vi "HTTP Request.vi"(0 "REST Client in":refnum<class "REST Client.lvclass">, 1 "Request body":string, 2 "Multipart Post data":T1[](array[typedef]), 5 "Method":T2, 9 "Path":string, 11 "error in (no error)":errorcluster, 12 "request specific headers":T3[](array[typedef]), 13 "timeout (0 = Use Default)":i32) -> (3 "Status Code":u16, 4 "REST Client out":refnum<class "REST Client.lvclass">, 6 "Response Headers out":refnum<class "Response Headers.lvclass">, 10 "Response body":string, 14 "Status String":string, 15 "error out":errorcluster)   [LabVIEW 2020, in "REST Client.lvlib" / "REST Client.lvclass"]
uses:
  REST Client.lvclass
  Response Headers/Response Headers.lvclass
  HTTP Header.ctl
  HTTP Methods.ctl
  <vilib>/httpClient/MultipartData.ctl
  <vilib>/NI/Advanced HTTP Client/Multipart Data--cluster.ctl
  <vilib>/VIPM Community/HTTP Client Plugin - Base/Classes/Abstract HTTP Client/Abstract HTTP Client.lvclass
  <vilib>/NI/Advanced HTTP Client/Session.lvclass
  http-client/http-client.lvclass
  <vilib>/httpClient/LabVIEWHTTPClient.lvlib
panel:
  # "Copyright © 2014 JKI All rights reserved.\n\nAuthor: Tomi Maila <tomi.maila@jki.net>\n\nThis library is provided \"AS IS\" ,WITHOUT WARRANTIES OR \nCONDITIONS OF ANY KIND, either express or implied.\n\nJKI -- jki.net"
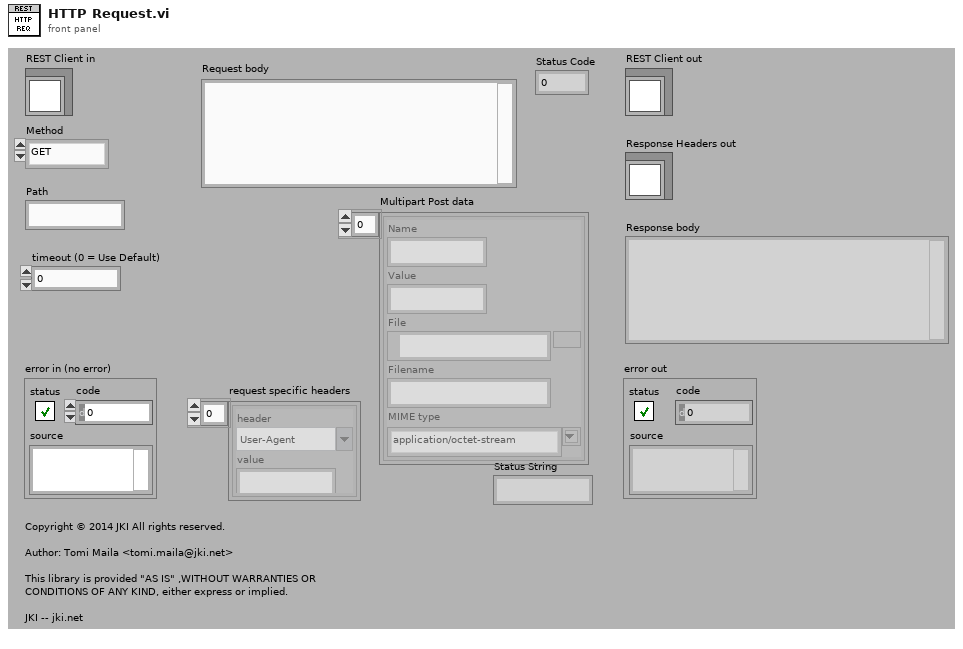
[diagram p1: front panel]
types:
  T1 = typedef "LabVIEWHTTPClient.lvlib/MultipartData.ctl" = cluster{"Name":string, "Value":string, "File":path, "Filename":string, "MIME type":string}
  T2 = typedef "REST Client.lvlib/REST Client.lvclass/HTTP Methods.ctl" = enum16{"GET", "HEAD", "POST", "PUT", "DELETE", "PATCH"}
  T3 = typedef "REST Client.lvlib/REST Client.lvclass/HTTP Header.ctl" = cluster{"header":string, "value":string}
  T4 = typedef "lib_NI_Advanced HTTP Client.lvlib/Session.lvclass/Multipart Data--cluster.ctl" = cluster{"name":string, "value":string, "file":path, "filename":string, "MIME type":string}
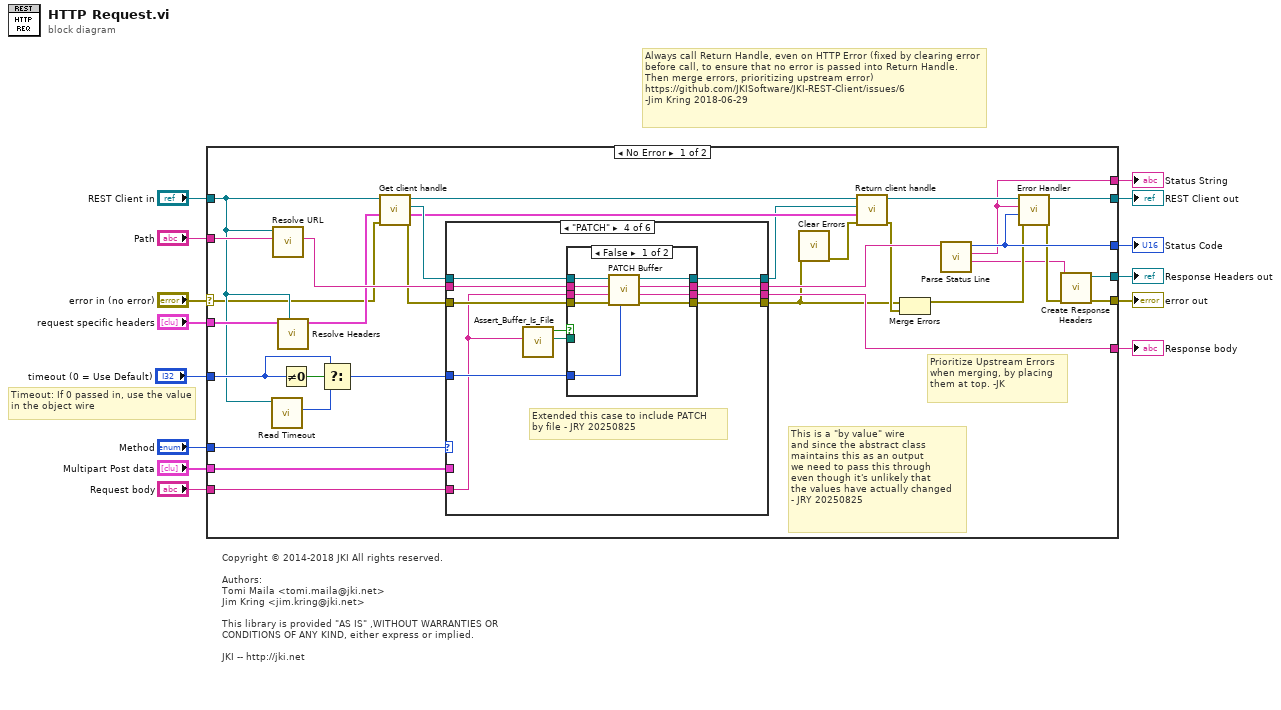
[diagram p0: block diagram]
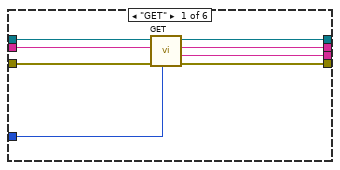
[diagram p2: hidden frame]
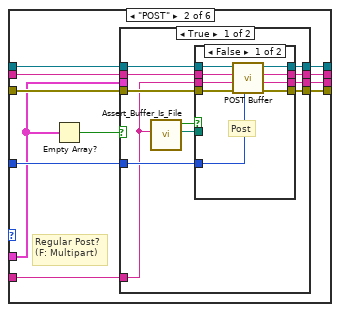
[diagram p3: hidden frame]
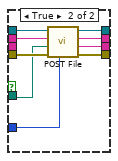
[diagram p4: hidden frame]
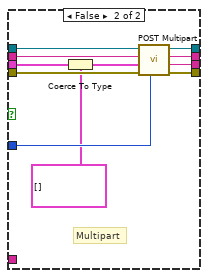
[diagram p5: hidden frame]
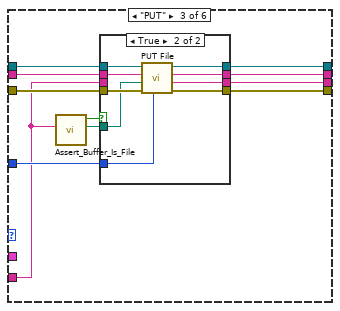
[diagram p6: hidden frame]
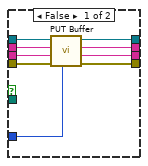
[diagram p7: hidden frame]
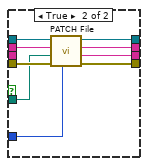
[diagram p8: hidden frame]
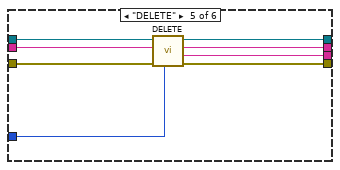
[diagram p9: hidden frame]
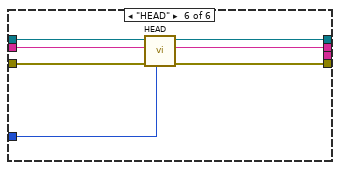
[diagram p10: hidden frame]
diagram:
  # "Always call Return Handle, even on HTTP Error (fixed by clearing error before call, to ensure that no error is passed into Return Handle. Then merge errors, prioritizing upstream error)\nhttps://github.com/JKISoftware/JKI-REST-Client/issues/6\n-Jim Kring 2018-06-29"
  # "Timeout: If 0 passed in, use the value in the object wire"
  # "Copyright © 2014-2018 JKI All rights reserved.\n\nAuthors:\nTomi Maila <tomi.maila@jki.net>\nJim Kring <jim.kring@jki.net>\n\nThis library is provided \"AS IS\" ,WITHOUT WARRANTIES OR \nCONDITIONS OF ANY KIND, either express or implied.\n\nJKI -- http://jki.net"
  n1 = case shown="No Error" "error in (no error)" {
    selector: "error in (no error)" -> [w15 w180]
    tunnel: [w34 w180] -> w13
    tunnel: [w41 w179] -> w11
    tunnel: "REST Client in" -> [w16 w179]
    tunnel: "Method" -> [w40 _]
    tunnel: "Path" -> [w39 _]
    tunnel: "Request body" -> [w26 _]
    tunnel: [w21 _] -> w8
    tunnel: [w35 _] -> w3
    tunnel: [w37 _] -> w7
    tunnel: "request specific headers" -> [w18 _]
    tunnel: [w36 _] -> w4
    tunnel: "Multipart Post data" -> [w33 _]
    tunnel: "timeout (0 = Use Default)" -> [w28 _]
    frame No Error {
      # "This is a \"by value\" wire\nand since the abstract class\nmaintains this as an output\nwe need to pass this through\neven though it's unlikely that\nthe values have actually changed\n- JRY 20250825"
      # "Prioritize Upstream Errors when merging, by placing them at top. -JK"
      n2 = call-dynamic "Read Timeout.vi"("REST Client in"=w16) -> ("Timeout"=w24:i32)  [unwired: 8 in, 2 out]
      n3 = call "Resolve URL.vi"("Path"=w39, "REST Client in"=w16) -> ("Resolved URL"=w38:string)  [unwired: 9 in]
      n4 = call "Resolve Headers.vi"("REST Client in"=w16, "headers in"=w18) -> ("headers out"=w17:T3[])  [unwired: 9 in]
      n5 = Not Equal To 0?(x=w28) -> (x != 0?=w29:bool)
      n6 = Select(t=w28, s=w29, f=w24) -> (s? t:f=w27:i32)
      n7 = call "Get client handle.vi"("error in (no error)"=w15, "headers"=w17, "REST Client in"=w16) -> ("error out"=w25:errorcluster, "headers out"=w43:T3[], "Client Handle"=w44:refnum<class "Abstract HTTP Client.lvclass">, "REST Client out"=w45:refnum<class "REST Client.lvclass">)  [unwired: 5 in]
      n8 = case shown="\"PATCH\"" w40 {
        tunnel: w38 -> [w53 w65 w116 w141 w166 w175]
        tunnel: w27 -> [w48 w64 w115 w142 w165 w177]
        tunnel: w25 -> [w52 w63 w114 w140 w170 w178]
        tunnel: [w49 w62 w113 w137 w167 w173] -> w46
        tunnel: [w50 w61 w112 w136 w168 _] -> w37
        tunnel: [w51 w60 w111 w135 w169 w176] -> w31
        tunnel: w44 -> [w54 w59 w110 w143 w171 w174]
        tunnel: w33 -> [_ w57 _ _ _ _]
        tunnel: w26 -> [_ w56 w109 w139 _ _]
        tunnel: [w47 w55 w106 w138 w164 w172] -> w19
        frame "GET" {
          n9 = call-dynamic "GET.vi"("timeout (10000)"=w48, "error in (no error)"=w52, "url"=w53, "HTTP Client Abstract in"=w54) -> ("error out"=w51:errorcluster, "body"=w50:string, "headers"=w49:string, "HTTP Client Abstract out"=w47:refnum<class "Abstract HTTP Client.lvclass">)  [unwired: 3 in, 1 out]
        }
        frame "POST" {
          # "Regular Post?\n(F: Multipart)"
          n10 = Empty Array?(array=w57) -> (empty?=w58:bool)
          n11 = case shown="True" w58 {
            tunnel: w65 -> [w76 w104]
            tunnel: w64 -> [w75 w99]
            tunnel: w63 -> [w74 w103]
            tunnel: [w73 w102] -> w62
            tunnel: [w72 w101] -> w61
            tunnel: [w71 w100] -> w60
            tunnel: w59 -> [w70 w105]
            tunnel: w56 -> [w69 _]
            tunnel: w57 -> [_ w96]
            tunnel: [w66 w95] -> w55
            frame True {
              n12 = call "Assert_Buffer_Is_File.vi"("body"=w69) -> ("File"=w67:path, "is File?"=w68:bool)  [unwired: 9 in]
              n13 = case shown="False" w68 {
                tunnel: w76 -> [w78 w89]
                tunnel: w75 -> [w81 w87]
                tunnel: w74 -> [w80 w90]
                tunnel: [w84 w93] -> w73
                tunnel: [w83 w92] -> w72
                tunnel: [w82 w91] -> w71
                tunnel: w70 -> [w85 w94]
                tunnel: w69 -> [w79 _]
                tunnel: w67 -> [_ w88]
                tunnel: [w77 w86] -> w66
                frame False {
                  # "Post"
                  n14 = call-dynamic "POST Buffer.vi"("timeout (10000)"=w81, "error in (no error)"=w80, "buffer"=w79, "url"=w78, "HTTP Client Abstract in"=w85) -> ("error out"=w82:errorcluster, "body"=w83:string, "headers"=w84:string, "HTTP Client Abstract out"=w77:refnum<class "Abstract HTTP Client.lvclass">)  [unwired: 2 in, 1 out]
                }
                frame True {
                  n15 = call-dynamic "POST File.vi"("timeout (10000)"=w87, "error in (no error)"=w90, "file"=w88, "url"=w89, "HTTP Client Abstract in"=w94) -> ("error out"=w91:errorcluster, "body"=w92:string, "headers"=w93:string, "HTTP Client Abstract out"=w86:refnum<class "Abstract HTTP Client.lvclass">)  [unwired: 2 in, 1 out]
                }
              }
            }
            frame False {
              # "Multipart"
              n16 = Coerce To Type(0:w96, 1:T4[] [] ("Multipart Post data")) -> (2:w97:T4[])
              n17 = call-dynamic "POST Multipart.vi"("timeout (10000)"=w99, "error in (no error)"=w103, "data"=w97, "url"=w104, "HTTP Client Abstract in"=w105) -> ("error out"=w100:errorcluster, "body"=w101:string, "headers"=w102:string, "HTTP Client Abstract out"=w95:refnum<class "Abstract HTTP Client.lvclass">)  [unwired: 2 in, 1 out]
            }
          }
        }
        frame "PUT" {
          n18 = call "Assert_Buffer_Is_File.vi"("body"=w109) -> ("File"=w107:path, "is File?"=w108:bool)  [unwired: 9 in]
          n19 = case shown="True" w108 {
            tunnel: w116 -> [w124 w127]
            tunnel: w115 -> [w121 w128]
            tunnel: w114 -> [w122 w133]
            tunnel: [w118 w130] -> w113
            tunnel: [w119 w131] -> w112
            tunnel: [w120 w132] -> w111
            tunnel: w110 -> [w125 w134]
            tunnel: w109 -> [w123 _]
            tunnel: w107 -> [_ w129]
            tunnel: [w117 w126] -> w106
            frame False {
              n20 = call-dynamic "PUT Buffer.vi"("timeout (10000)"=w121, "error in (no error)"=w122, "buffer"=w123, "url"=w124, "HTTP Client Abstract in"=w125) -> ("error out"=w120:errorcluster, "body"=w119:string, "headers"=w118:string, "HTTP Client Abstract out"=w117:refnum<class "Abstract HTTP Client.lvclass">)  [unwired: 2 in, 1 out]
            }
            frame True {
              n21 = call-dynamic "PUT File.vi"("timeout (10000)"=w128, "error in (no error)"=w133, "file"=w129, "url"=w127, "HTTP Client Abstract in"=w134) -> ("error out"=w132:errorcluster, "body"=w131:string, "headers"=w130:string, "HTTP Client Abstract out"=w126:refnum<class "Abstract HTTP Client.lvclass">)  [unwired: 2 in, 1 out]
            }
          }
        }
        frame "PATCH" {
          # "Extended this case to include PATCH\nby file - JRY 20250825"
          n22 = call "Assert_Buffer_Is_File.vi"("body"=w139) -> ("File"=w144:path, "is File?"=w145:bool)  [unwired: 9 in]
          n23 = case shown="False" w145 {
            tunnel: w141 -> [w153 w156]
            tunnel: w142 -> [w150 w157]
            tunnel: w140 -> [w151 w162]
            tunnel: [w147 w159] -> w137
            tunnel: [w148 w160] -> w136
            tunnel: [w149 w161] -> w135
            tunnel: w143 -> [w154 w163]
            tunnel: w139 -> [w152 _]
            tunnel: w144 -> [_ w158]
            tunnel: [w146 w155] -> w138
            frame False {
              n24 = call-dynamic "PATCH Buffer.vi"("timeout"=w150, "error in (no error)"=w151, "buffer"=w152, "url"=w153, "HTTP Client Abstract in"=w154) -> ("error out"=w149:errorcluster, "body"=w148:string, "headers"=w147:string, "HTTP Client Abstract out"=w146:refnum<class "Abstract HTTP Client.lvclass">)  [unwired: 2 in, 1 out]
            }
            frame True {
              n25 = call-dynamic "PATCH File.vi"("timeout"=w157, "error in (no error)"=w162, "file"=w158, "url"=w156, "HTTP Client Abstract in"=w163) -> ("error out"=w161:errorcluster, "body"=w160:string, "headers"=w159:string, "HTTP Client Abstract out"=w155:refnum<class "Abstract HTTP Client.lvclass">)  [unwired: 2 in, 1 out]
            }
          }
        }
        frame "DELETE" {
          n26 = call-dynamic "DELETE.vi"("timeout (10000)"=w165, "error in (no error)"=w170, "url"=w166, "HTTP Client Abstract in"=w171) -> ("error out"=w169:errorcluster, "body"=w168:string, "headers"=w167:string, "HTTP Client Abstract out"=w164:refnum<class "Abstract HTTP Client.lvclass">)  [unwired: 3 in, 1 out]
        }
        frame "HEAD" {
          n27 = call-dynamic "HEAD.vi"("timeout (10000)"=w177, "error in (no error)"=w178, "url"=w175, "HTTP Client Abstract in"=w174) -> ("error out"=w176:errorcluster, "headers"=w173:string, "HTTP Client Abstract out"=w172:refnum<class "Abstract HTTP Client.lvclass">)  [unwired: 4 in, 1 out]
        }
      }
      n28 = call <vilib>:"Clear Errors.vi"("error in (no error)"=w31) -> ("error out"=w30:errorcluster)  [unwired: 5 in, 1 out]
      n29 = call "Return client handle.vi"("error in (no error)"=w30, "headers"=w43, "Client Handle"=w19, "REST Client in"=w45) -> ("error out"=w32:errorcluster, "REST Client out"=w42:refnum<class "REST Client.lvclass">)  [unwired: 6 in]
      n30 = Merge Errors(w31, w32) -> (w22:errorcluster)
      n31 = call "Parse Status Line.vi"("Headers w/ status line"=w46) -> ("HTTP Headers"=w20:string, "Status String"=w21:string, "status code"=w36:u16)  [unwired: 6 in, 2 out]
      n32 = call-dynamic "Error Handler.vi"("error in (no error)"=w22, "Status Code"=w36, "Status String"=w21, "REST Client in"=w42) -> ("error out"=w23:errorcluster, "REST Client out"=w41:refnum<class "REST Client.lvclass">)  [unwired: 6 in]
      n33 = call "Create Response Headers.vi"("error in (no error)"=w23, "Response Headers"=w20) -> ("error out"=w34:errorcluster, "Response Headers out"=w35:refnum<class "Response Headers.lvclass">)  [unwired: 8 in]
    }
    frame Error {
    }
  }
  "error out" <- w13
  "REST Client out" <- w11
  "Status Code" <- w4
  "Status String" <- w8
  "Response Headers out" <- w3
  "Response body" <- w7
